vi "Subscribe.vi"(6 "Time out (ms)":i32=1000, 7 "Topic":string, 8 "error in (no error)":errorcluster, 9 "WAMP Client in":refnum<class "WAMP Client.lvclass">) -> (0 "Publication Received Event":refnum<user-event>, 1 "Success?":bool, 2 "error out":errorcluster, 3 "WAMP Client out":refnum<class "WAMP Client.lvclass">)   [LabVIEW 2020, in "WAMP Client.lvclass"]
uses:
  <userlib>/lvwamp/WAMP Client/WAMP Client.lvclass
  <vilib>/ErrorRing/Error Ring.xnode
  <vilib>/Utility/error.llb/Error Cluster From Error Code.vi
  <userlib>/lvwamp/WAMP Client/TypeDef/EVENT Payload.ctl
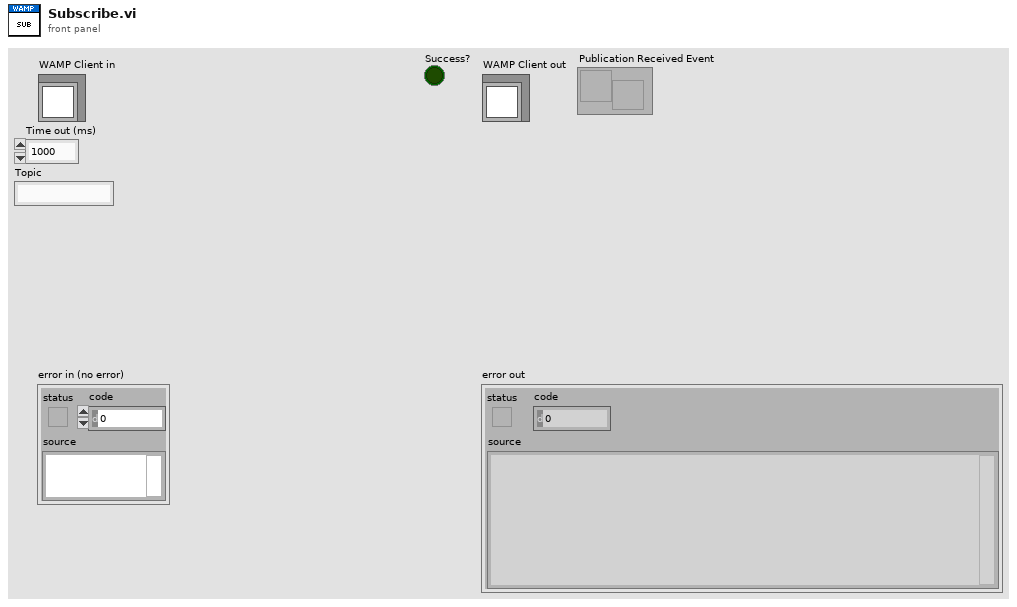
[diagram p1: front panel]
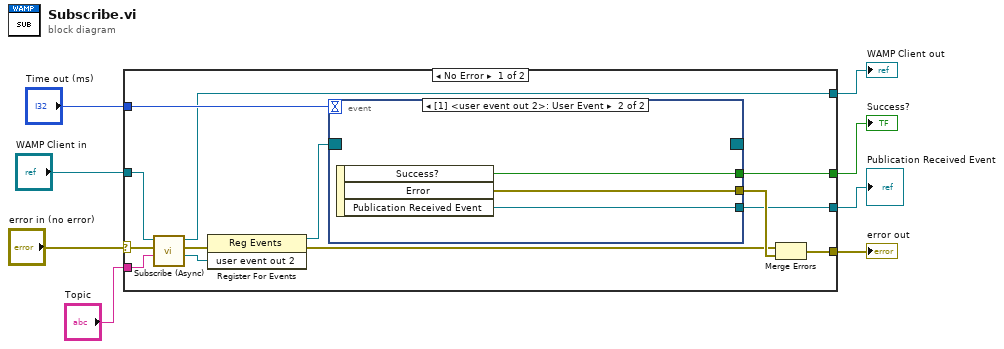
[diagram p0: block diagram]
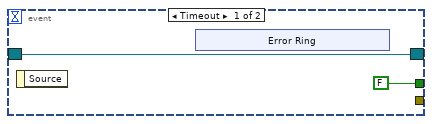
[diagram p2: hidden frame]
diagram:
  n1 = case shown="No Error" "error in (no error)" {
    selector: "error in (no error)" -> [w16 w33]
    tunnel: [w10 w33] -> w8
    tunnel: [w13 w32] -> w6
    tunnel: "WAMP Client in" -> [w18 w32]
    tunnel: [w20 _] -> w5
    tunnel: "Time out (ms)" -> [w19 _]
    tunnel: "Topic" -> [w17 _]
    tunnel: [w9 _] -> w1
    frame No Error {
      n2 = call-dynamic "Subscribe (Async).vi"("Topic"=w17, "error in (no error)"=w16, "WAMP Client in"=w18) -> ("user event out 2"=w15:refnum<user-event>, "error out"=w14:errorcluster, "WAMP Client out"=w13:refnum<class "WAMP Client.lvclass">)  [unwired: 6 in]
      n3 = register-events(error in=w14, w15) -> (reference out=w21:refnum<event-registration>, error out=w11:errorcluster)  [unwired: 1 in]
      n4 = event shown="[1] <user event out 2>: User Event" {
        selector: w21 -> [w22 _]
        dyn-events: [w22 _] -> _
        timeout: w19 -> [_ _]
        tunnel: [FALSE ("Success?") w31] -> w20
        tunnel: [_ w30] -> w12
        tunnel: [_ w29] -> w9
        event Timeout {
          n5 = event-data() -> ()  [unwired: 1 in, 1 out]
          n6 = xnode "Error Ring"() -> ()  [unwired: 1 out]
        }
        event User Event {
          n7 = event-data() -> ("Success?"=w31:bool, "Error"=w30:errorcluster, "Publication Received Event"=w29:refnum<user-event>)  [unwired: 1 in]
        }
      }
      n8 = Merge Errors(w11, w12) -> (w10:errorcluster)
    }
    frame Error {
    }
  }
  "error out" <- w8
  "WAMP Client out" <- w6
  "Success?" <- w5
  "Publication Received Event" <- w1
